vi "Get Image Percentiles.vi"(6 "Update needed":bool, 8 "error in (no error)":errorcluster, 9 "Low Percentile (0-100)":dbl min=0.0 max=100.0, 10 "High Percentile (0-100)":dbl min=0.0 max=100.0, 11 "Image in":T1) -> (0 "error out":errorcluster, 1 "Low percentile Value":sgl, 2 "High percentile Value":sgl)   [LabVIEW 2021, in "Image.lvlib"]
uses:
  Image.lvlib
  <vilib>/vision/Image Controls.llb/IMAQ Image.ctl
  51996c9b-8f8a-4421-b785-6f756e70cddc.vi
  f93208cd-6e65-4f11-8911-6a85aabe3361.vi
  <vilib>/vision/EDVR.llb/IMAQ ImageToEDVR 2D U8.vi
  <vilib>/vision/EDVR.llb/IMAQ ImageToEDVR 2D I16.vi
  <vilib>/vision/EDVR.llb/IMAQ ImageToEDVR 2D SGL.vi
  <vilib>/vision/EDVR.llb/IMAQ ImageToEDVR 2D U16.vi
  <vilib>/Utility/error.llb/Error Cluster From Error Code.vi
  <userlib>/_OpenG.lib/array/array.llb/Index Array Elements__ogtk.vi
  <userlib>/_OpenG.lib/array/array.llb/Index 1D Array Elements (SGL)__ogtk.vi
  <vilib>/ErrorRing/Error Ring.xnode
panel:
  out "changed or first call?":bool
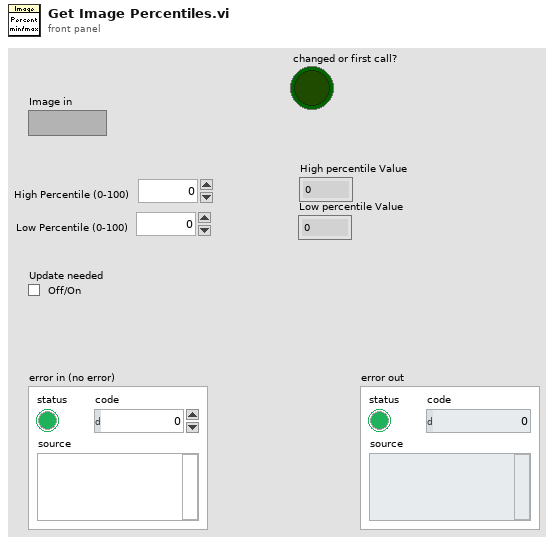
[diagram p1: front panel]
types:
  T1 = typedef "IMAQ Image.ctl" = refnum<image>
  T2 = typedef "Image Type" = u32
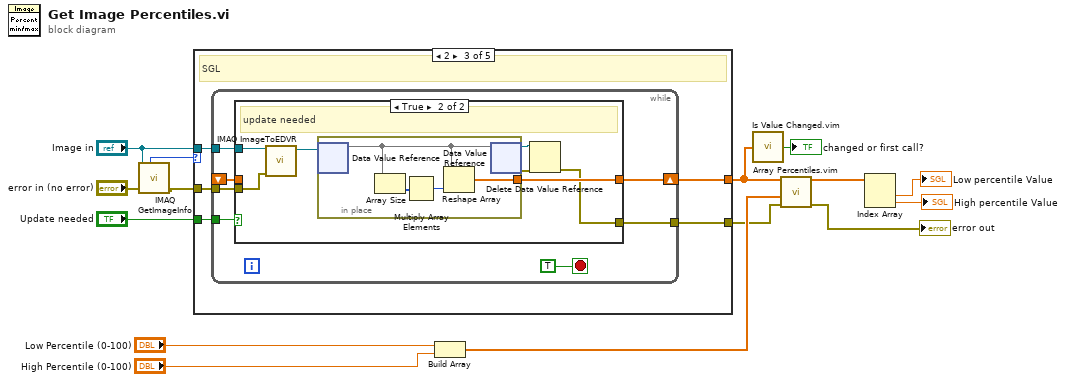
[diagram p0: block diagram]
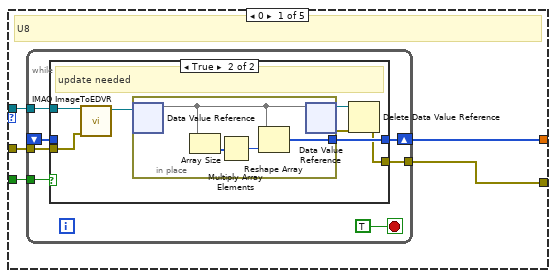
[diagram p2: hidden frame]
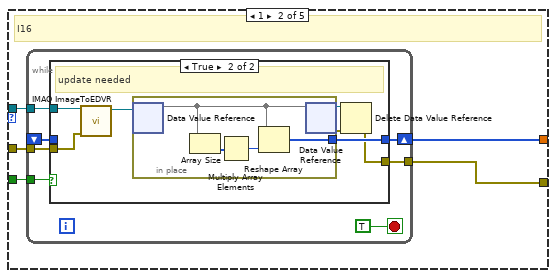
[diagram p4: hidden frame]
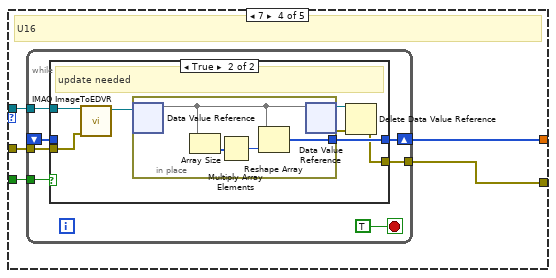
[diagram p7: hidden frame]
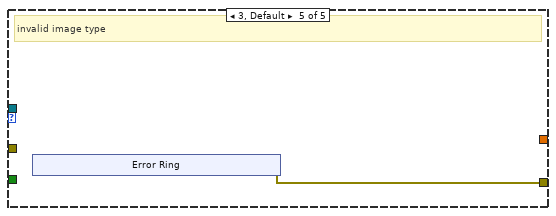
[diagram p9: hidden frame]
diagram:
  n1 = call "IMAQ GetImageInfo"("error in (no error)"="error in (no error)", "Image"="Image in") -> ("error out"=w14:errorcluster, "Image Type"=w13:T2)  [unwired: 2 in, 6 out]
  n2 = case shown="2" w13 {
    tunnel: w14 -> [w19 w44 w69 w94 _]
    tunnel: "Image in" -> [w20 w45 w70 w95 _]
    tunnel: [w17 w41 w66 w91 w116] -> w4
    tunnel: "Update needed" -> [w18 w43 w68 w93 _]
    tunnel: [w16 w42 w67 w92 _] -> w2
    frame 0 {
      # "U8"
      n3 = while {
        tunnel: w20 -> [w27]
        tunnel: w19 -> [w26]
        tunnel: [w25] -> w17
        shift-right: [w24] -> w16
        shift-left: _ -> [w22]
        tunnel: w18 -> [w21]
        stop <- TRUE stop-if-true
        n4 = case shown="True" w21 {
          tunnel: w27 -> [_ w36]
          tunnel: w26 -> [w29 w35]
          tunnel: [w29 w30] -> w25
          tunnel: [w28 w33] -> w24
          tunnel: w22 -> [w28 _]
          frame False {
            # "no update needed"
          }
          frame True {
            # "update needed"
            n5 = call-poly <vilib>:"IMAQ ImageToEDVR.vi"("error in (no error)"=w35, "Image"=w36) -> ("EDVR 2D U8"=w34:refnum<data-value>)  [unwired: 7 in, 2 out]
            n6 = in-place {
              in-place-border: [w37] -> w33
              n7 = in-place-dvr #1(w34) -> (w38:u8[][])  [unwired: 1 out]
              n8 = Array Size(array=w38) -> (size(s)=w40:i32[])
              n9 = Multiply Array Elements(1:w40) -> (0:w39:i32)
              n10 = Reshape Array(w38, w39) -> (w37:u8[])
              n11 = in-place-dvr #1(w38) -> (w32:refnum<data-value>, w31:errorcluster)
            }
            n12 = Delete Data Value Reference(data value reference=w32, error in=w31) -> (error out=w30:errorcluster)  [unwired: 1 out]
          }
        }
      }
    }
    frame 1 {
      # "I16"
      n13 = while {
        tunnel: w45 -> [w52]
        tunnel: w44 -> [w51]
        tunnel: [w50] -> w41
        shift-right: [w49] -> w42
        shift-left: _ -> [w47]
        tunnel: w43 -> [w46]
        stop <- TRUE stop-if-true
        n14 = case shown="True" w46 {
          tunnel: w52 -> [_ w61]
          tunnel: w51 -> [w54 w60]
          tunnel: [w54 w55] -> w50
          tunnel: [w53 w58] -> w49
          tunnel: w47 -> [w53 _]
          frame False {
            # "no update needed"
          }
          frame True {
            # "update needed"
            n15 = call-poly <vilib>:"IMAQ ImageToEDVR.vi"("error in (no error)"=w60, "Image"=w61) -> ("EDVR 2D I16"=w59:refnum<data-value>)  [unwired: 7 in, 2 out]
            n16 = in-place {
              in-place-border: [w62] -> w58
              n17 = in-place-dvr #2(w59) -> (w63:i16[][])  [unwired: 1 out]
              n18 = Array Size(array=w63) -> (size(s)=w65:i32[])
              n19 = Multiply Array Elements(1:w65) -> (0:w64:i32)
              n20 = Reshape Array(w63, w64) -> (w62:i16[])
              n21 = in-place-dvr #2(w63) -> (w57:refnum<data-value>, w56:errorcluster)
            }
            n22 = Delete Data Value Reference(data value reference=w57, error in=w56) -> (error out=w55:errorcluster)  [unwired: 1 out]
          }
        }
      }
    }
    frame 2 {
      # "SGL"
      n23 = while {
        tunnel: w70 -> [w77]
        tunnel: w69 -> [w76]
        tunnel: [w75] -> w66
        shift-right: [w74] -> w67
        shift-left: _ -> [w72]
        tunnel: w68 -> [w71]
        stop <- TRUE stop-if-true
        n24 = case shown="True" w71 {
          tunnel: w77 -> [_ w86]
          tunnel: w76 -> [w79 w85]
          tunnel: [w79 w80] -> w75
          tunnel: [w78 w83] -> w74
          tunnel: w72 -> [w78 _]
          frame False {
            # "no update needed"
          }
          frame True {
            # "update needed"
            n25 = call-poly <vilib>:"IMAQ ImageToEDVR.vi"("error in (no error)"=w85, "Image"=w86) -> ("EDVR 2D SGL"=w84:refnum<data-value>)  [unwired: 7 in, 2 out]
            n26 = in-place {
              in-place-border: [w87] -> w83
              n27 = in-place-dvr #3(w84) -> (w88:sgl[][])  [unwired: 1 out]
              n28 = Array Size(array=w88) -> (size(s)=w90:i32[])
              n29 = Multiply Array Elements(1:w90) -> (0:w89:i32)
              n30 = Reshape Array(w88, w89) -> (w87:sgl[])
              n31 = in-place-dvr #3(w88) -> (w82:refnum<data-value>, w81:errorcluster)
            }
            n32 = Delete Data Value Reference(data value reference=w82, error in=w81) -> (error out=w80:errorcluster)  [unwired: 1 out]
          }
        }
      }
    }
    frame 7 {
      # "U16"
      n33 = while {
        tunnel: w95 -> [w102]
        tunnel: w94 -> [w101]
        tunnel: [w100] -> w91
        shift-right: [w99] -> w92
        shift-left: _ -> [w97]
        tunnel: w93 -> [w96]
        stop <- TRUE stop-if-true
        n34 = case shown="True" w96 {
          tunnel: w102 -> [_ w111]
          tunnel: w101 -> [w104 w110]
          tunnel: [w104 w105] -> w100
          tunnel: [w103 w108] -> w99
          tunnel: w97 -> [w103 _]
          frame False {
            # "no update needed"
          }
          frame True {
            # "update needed"
            n35 = call-poly <vilib>:"IMAQ ImageToEDVR.vi"("error out"=w110, "Image"=w111) -> ("EDVR 2D U16"=w109:refnum<data-value>)  [unwired: 7 in, 2 out]
            n36 = in-place {
              in-place-border: [w112] -> w108
              n37 = in-place-dvr #4(w109) -> (w113:u16[][])  [unwired: 1 out]
              n38 = Array Size(array=w113) -> (size(s)=w115:i32[])
              n39 = Multiply Array Elements(1:w115) -> (0:w114:i32)
              n40 = Reshape Array(w113, w114) -> (w112:u16[])
              n41 = in-place-dvr #4(w113) -> (w107:refnum<data-value>, w106:errorcluster)
            }
            n42 = Delete Data Value Reference(data value reference=w107, error in=w106) -> (error out=w105:errorcluster)  [unwired: 1 out]
          }
        }
      }
    }
    frame 3, Default {
      # "invalid image type"
      n43 = xnode "Error Ring"() -> ("error out"=w116:errorcluster)
    }
  }
  n44 = Build Array("Low Percentile (0-100)", "High Percentile (0-100)") -> (w5:dbl[])
  n45 = call "Is Value Changed.vim"("value"=w2) -> ("changed or first call?"=→"changed or first call?":bool)
  n46 = call "Array Percentiles.vim"("Error In"=w4, "Percentile Array"=w5, "Array"=w2) -> ("Error Out"=→"error out":errorcluster, "percentiles"=w6:sgl[])  [unwired: 7 in]
  n47 = Index Array(array=w6) -> (element #1=→"Low percentile Value":sgl, element #2=→"High percentile Value":sgl)  [unwired: 2 in]
